vi "Set Property.vi"(10 "Ctl Ref":refnum<vi>, 11 "UIP In":refnum<class "UIP Interface.lvclass">) -> (0 "Error Out":errorcluster, 3 "UIP Out":refnum<class "UIP Interface.lvclass">)   [LabVIEW 2020, in "UIM.lvlib" / "UIP Interface.lvclass"]
doc: "Overwrite this abstract method to implement child behavior for applying UIP private data into the VI Server Control property."
uses:
  UIP Interface/UIP Interface.lvclass
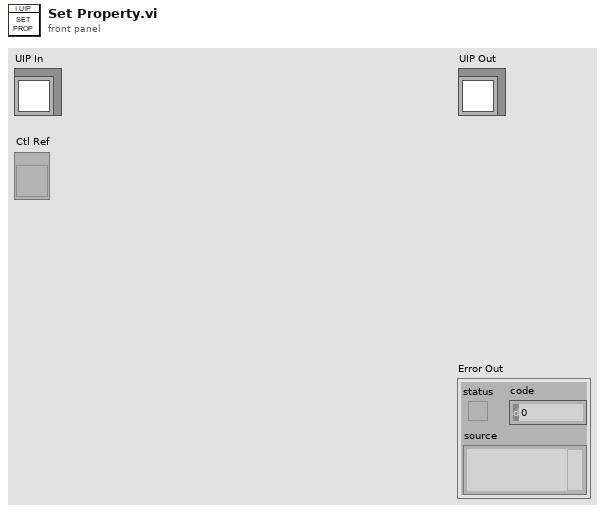
[diagram p1: front panel]
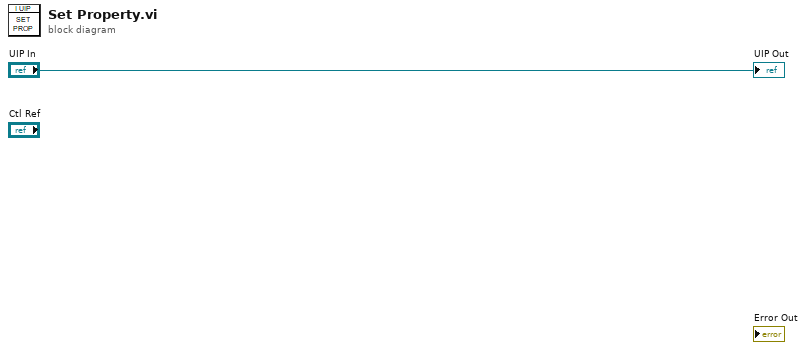
[diagram p0: block diagram]
diagram:
  "UIP Out" <- "UIP In"
